vi "MinMaxScaler.vi"(8 "error in (no error)":errorcluster caption="entrée d'erreur (pas d'erreur)", 11 "MinMaxScaler":T1={"feature_range"={"min"=0.0, "max"=1.0}, "copy"=TRUE}) -> (0 "error out":errorcluster, 3 "MinMaxScaler.lvclass":refnum<class "MinMaxScaler.lvclass">)   [LabVIEW 2020]
doc: "Transform features by scaling each feature to a given range.\n\nThis estimator scales and translates each feature individually such that it is in the given range on the training set, e.g. between zero and one.\n\nThe transformation is given by:\n\nX_std = (X - X.min(axis=0)) / (X.max(axis=0) - X.min(axis=0))\nX_scaled = X_std * (max - min) + min\nwhere min, max = feature_range.\n\nThis transformation is often used as an alternative to zero mean, unit variance scaling.\n\n\nParameters : \n\n- feature_range : tuple (min, max), default=(0, 1)\nDesired range of transformed data.\n\n- copy : bool, default=True\nSet to False to perform inplace row normalization and avoid a copy (if the input is already a numpy array).\n\n\n\nMethods : \n\n- Fit : Compute the minimum and maximum to be used for later scaling.\n\nParameters : X : array-like of shape (n_samples, n_features)\n The data used to compute the per-feature minimum and maximum used for later scaling along the features axis.\n y : None\n Ignored.\n\n\n- Fit Transform : Fit to data, then transform it. Fits transformer to X and y with optional parameters fit_params and returns a transformed version of X.\n\nParameters : X : {array-like, sparse matrix, dataframe} of shape (n_samples, n_features)\n y : ndarray of shape (n_samples,), default=None\n Target values.\n\nReturns : X_new : ndarray array of shape (n_samples, n_features_new)\n Transformed array.\n\n\n- Partial Fit : Online computation of min and max on X for later scaling. All of X is processed as a single batch. This is intended for cases when fit is not feasible due to very large number of n_samples or because X is read from a continuous stream.\n\nParameters : X : array-like of shape (n_samples, n_features)\n The data used to compute the mean and standard deviation used for later scaling along the features axis.\n y : None\n Ignored.\n\n\n- Transform : Scale features of X according to feature_range.\n\nParameters : X : array-like of shape (n_samples, n_features)\n Input data that will be transformed.\n\nReturns : Xt : array-like of shape (n_samples, n_features)\n Transformed data."
uses:
  MinMaxScaler.lvclass
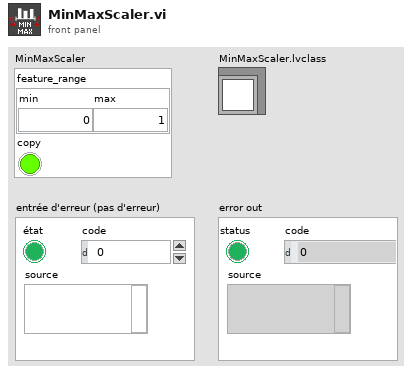
[diagram p1: front panel]
types:
  T1 = cluster{"feature_range":cluster{"min":dbl, "max":dbl}, "copy":bool}
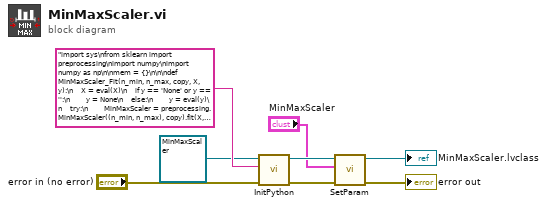
[diagram p0: block diagram]
diagram:
  n1 = call-dynamic "InitPython.vi"("error in (no error)"="error in (no error)", "Python Instruction"="import sys\nfrom sklearn import preprocessing\nimport numpy\nimport numpy as np\n\nmem = {}\n\n\ndef MinMaxScaler_Fit(n_min, n_max, copy, X, y):\n    X = eval(X)\n    if y == 'None' or y == '':\n        y = None\n    else:\n        y = eval(y)\n    try:\n        MinMaxScaler = preprocessing.MinMaxScaler((n_min, n_max), copy).fit(X, y)\n        mem['FitMinMaxScaler'] = MinMaxScaler\n        return str('OK')\n    except:\n        erreur = sys.exc_info()\n        typerr = u\"%s\" % (erreur[0])\n        typerr = typerr[typerr.find(\"'\")+1:typerr.rfind(\"'\")]\n        msgerr = u\"%s\" % (erreur[1])\n        message = str('/!\\\\ {0} : {1}'. format(typerr,msgerr))\n        return message \n    \ndef MinMaxScaler_FitTransform(n_min, n_max, copy, X, y):\n    X = eval(X)\n    if y == 'None' or y == '':\n        y = None\n    else:\n        y = eval(y)\n    try:\n        MinMaxScaler = preprocessing.MinMaxScaler((n_min, n_max), copy).fit_transform(X, y)\n        dtype = type(MinMaxScaler)\n        if dtype == numpy.ndarray:\n            MinMaxScaler = MinMaxScaler.tolist()\n            return str(MinMaxScaler) \n        else:\n            Mat = MinMaxScaler.tocoo()\n            return str(list(zip(Mat.row, Mat.col, Mat.data)))\n    except:\n        erreur = sys.exc_info()\n        typerr = u\"%s\" % (erreur[0])\n        typerr = typerr[typerr.find(\"'\")+1:typerr.rfind(\"'\")]\n        msgerr = u\"%s\" % (erreur[1])\n        message = str('/!\\\\ {0} : {1}'. format(typerr,msgerr))\n        return message \n\ndef MinMaxScaler_Transform(n_min, n_max, copy, X, y):\n    X = eval(X)\n    if y == 'None' or y == '':\n        y = None\n    else:\n        y = eval(y)\n    try:\n        MinMaxScaler = mem['FitMinMaxScaler'].transform(X)\n        dtype = type(MinMaxScaler)\n        if dtype == numpy.ndarray:\n            MinMaxScaler = MinMaxScaler.tolist()\n            return str(MinMaxScaler) \n        else:\n            Mat = MinMaxScaler.tocoo()\n            return str(list(zip(Mat.row, Mat.col, Mat.data)))\n    except:\n        erreur = sys.exc_info()\n        typerr = u\"%s\" % (erreur[0])\n        typerr = typerr[typerr.find(\"'\")+1:typerr.rfind(\"'\")]\n        msgerr = u\"%s\" % (erreur[1])\n        message = str('/!\\\\ {0} : {1}'. format(typerr,msgerr))\n        return message\n    \ndef MinMaxScaler_Partial_Fit(n_min, n_max, copy, X, y):\n    X = eval(X)\n    if y == 'None' or y == '':\n        y = None\n    else:\n        y = eval(y)\n    try:\n        MinMaxScaler = preprocessing.MinMaxScaler((n_min, n_max), copy).partial_fit(X, y)\n        mem['FitMinMaxScaler'] = MinMaxScaler\n        return str('OK')\n    except:\n        erreur = sys.exc_info()\n        typerr = u\"%s\" % (erreur[0])\n        typerr = typerr[typerr.find(\"'\")+1:typerr.rfind(\"'\")]\n        msgerr = u\"%s\" % (erreur[1])\n        message = str('/!\\\\ {0} : {1}'. format(typerr,msgerr))\n        return message", "Scikit-learn en entrée"=refnum<class "MinMaxScaler.lvclass"> refnum ("MinMaxScaler.lvclass")) -> ("error out"=w2:errorcluster, "Scikit-learn en sortie"=w5:refnum<class "MinMaxScaler.lvclass">)  [unwired: 7 in]
  n2 = call-dynamic "SetParam.vi"("error in (no error)"=w2, "MinMaxScaler"="MinMaxScaler", "MinMaxScaler.lvclass"=w5) -> ("error in (no error)"=→"error out":errorcluster, "MinMaxScaler.lvclass"=→"MinMaxScaler.lvclass":refnum<class "MinMaxScaler.lvclass">)  [unwired: 7 in]
